vi "SR400_settings_monitoring.vi"(0 "Count Time Set":dbl[unit]=0.01, 1 "# of periods (def: 1)":i32=1, 3 "j (0)":T1, 4 "Scan End Mode (Def: Stop)":enum16{"Stop", "Start"}(ring), 5 "VISA_SR400":refnum<visa-resource-name>="GPIB0::23::INSTR") -> (2 "VISA resource name out":refnum<visa-resource-name>)   [LabVIEW 2015]
uses:
  Libraries/SR400/Public/Typedefs/Output Scale.ctl
  Libraries/SR400/Public/Typedefs/Counter.ctl
  Libraries/SR400/Public/Typedefs/Output Source.ctl
  Libraries/SR400/SR400.lvlib
panel:
  out "errorOUT":errorcluster caption="Error Out"
  out "ttimeOUT":dbl[unit]=1.0 caption="Count Time Current" min=0.0 max=10000.0 step=1.0 format="%#_7g"
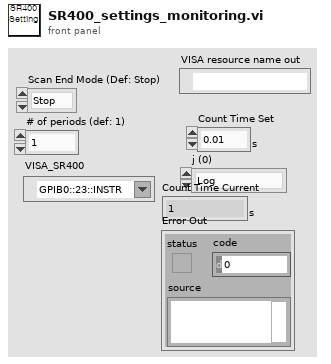
[diagram p1: front panel]
types:
  T1 = typedef "SR400.lvlib/Output Scale.ctl" = enum16{"Log", "987######", "#876#####", "##765####", "###654###", "####543##", "#####432#", "######321"}
  T2 = typedef "SR400.lvlib/Output Source.ctl" = enum16{"A", "B", "A - B", "A + B"}
  T3 = typedef "SR400.lvlib/Counter.ctl" = enum16{"Counter A", "Counter B", "Counter T"}
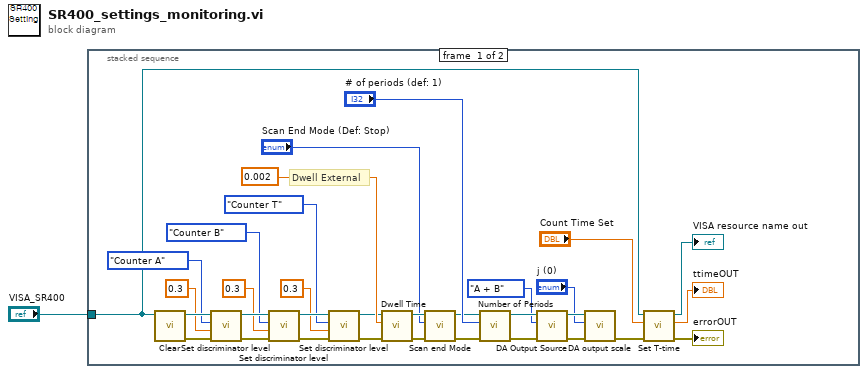
[diagram p0: block diagram]
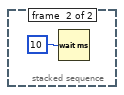
[diagram p2: hidden frame]
diagram:
  n1 = stacked-sequence {
    tunnel: "VISA_SR400" -> [w6 _]
    frame #0 {
      # "Dwell External"
      n2 = call "Clear.vi"("VISA resource name"=w6) -> ("error out"=w21:errorcluster, "VISA resource name out"=w34:refnum<visa-resource-name>)  [unwired: 9 in]
      n3 = call "Set discriminator level.vi"("error in (no error)"=w21, "Level (-0.034 V)"=0.3, "Discriminator (def: A)"=Counter."Counter A", "VISA resource name"=w34) -> ("error out"=w20:errorcluster, "VISA resource name out"=w31:refnum<visa-resource-name>)  [unwired: 6 in]
      n4 = call "Set discriminator level.vi"("error in (no error)"=w20, "Level (-0.034 V)"=0.3, "Discriminator (def: A)"=Counter."Counter B", "VISA resource name"=w31) -> ("error out"=w19:errorcluster, "VISA resource name out"=w28:refnum<visa-resource-name>)  [unwired: 6 in]
      n5 = call "Set discriminator level.vi"("error in (no error)"=w19, "Level (-0.034 V)"=0.3, "Discriminator (def: A)"=Counter."Counter T", "VISA resource name"=w28) -> ("error out"=w16:errorcluster, "VISA resource name out"=w17:refnum<visa-resource-name>)  [unwired: 6 in]
      n6 = call "Dwell Time.vi"("error in (no error)"=w16, "Dwell time (0.002 s)"=0.002, "VISA resource name"=w17) -> ("error out"=w18:errorcluster, "VISA resource name out"=w24:refnum<visa-resource-name>)  [unwired: 7 in]
      n7 = call "Scan end Mode.vi"("error in (no error)"=w18, "Scan End Mode (Def: Stop)"="Scan End Mode (Def: Stop)", "VISA resource name"=w24) -> ("error out"=w14:errorcluster, "VISA resource name out"=w15:refnum<visa-resource-name>)  [unwired: 7 in]
      n8 = call "Number of Periods.vi"("error in (no error)"=w14, "# of periods (def: 1)"="# of periods (def: 1)", "VISA resource name"=w15) -> ("error out"=w12:errorcluster, "VISA resource name out"=w13:refnum<visa-resource-name>)  [unwired: 7 in]
      n9 = call "DA Output Source.vi"("error in (no error)"=w12, "j (0)"=Output_Source."A + B", "VISA resource name"=w13) -> ("error out"=w9:errorcluster, "VISA resource name out"=w10:refnum<visa-resource-name>)  [unwired: 7 in]
      n10 = call "DA output scale.vi"("error in (no error)"=w9, "j (0)"="j (0)", "VISA resource name"=w10) -> ("error out"=w7:errorcluster)  [unwired: 7 in, 1 out]
      n11 = call "Set T-time.vi"("errorIN"=w7, "Count Time Set"="Count Time Set", "VISA resource name"=w6) -> ("errorOUT"=→"errorOUT":errorcluster, "ttimeOUT"=→"ttimeOUT":dbl[unit], "VISA resource name out"=→"VISA resource name out":refnum<visa-resource-name>)  [unwired: 4 in]
    }
    frame #1 {
      n12 = Wait (ms)(milliseconds to wait=u32 10) -> ()  [unwired: 1 out]
    }
  }
